vi "Teleop.vi"(10 "Match Info":T1={"Autonomous Elapsed Seconds"=0.0, "TeleOp Elapsed Seconds"=0.0, "Disabled Elapsed Seconds"=0.0, "Visited Autonomous"=FALSE, "Visited TeleOp"=FALSE, "Visited Disabled"=FALSE, "Autonomous Settings"={"Autonomous Style"=enum."Independent", "VI Refnum"=refnum}}, 11 "Call Context":T2) -> ()   [LabVIEW 2015]
doc: "This VI is called for each TeleOp packet received from the DS where the robot is not disabled. It is often used to read from the joysticks and update I/O or to update setpoints for timed control loops. It should complete and return within 20 milliseconds or it may miss DS packets."
uses:
  <vilib>/Rock Robotics/WPI/DriverStation/WPI_DriverStationDerivedRobotMode.ctl
  <vilib>/Rock Robotics/WPI/DriverStation/WPI_DriverStationMatch Info.ctl
  <vilib>/Rock Robotics/WPI/Solenoid/WPI_SolenoidValue.ctl
  <vilib>/Rock Robotics/WPI/Utilities/WPI_GetSetVariantRefNum.vi
  <vilib>/Rock Robotics/Network Tables/NT Write Boolean Array.vi
  <vilib>/Rock Robotics/Network Tables/NT Write Numeric Array.vi
  <vilib>/Rock Robotics/Network Tables/NT Read Boolean.vi
  <vilib>/Rock Robotics/Network Tables/NT Read Number.vi
  <vilib>/Rock Robotics/WPI/Solenoid/WPI_SolenoidSetEnum.vi
  <vilib>/Rock Robotics/Network Tables/NT Write Number.vi
panel:
  out "Compressor Running":bool
  out "Enabled":bool
  out "Sample Slider 0":dbl(slide) scale=0.0..5.0
  out "Sample Boolean 1":bool
  out "Sample Boolean 0":bool
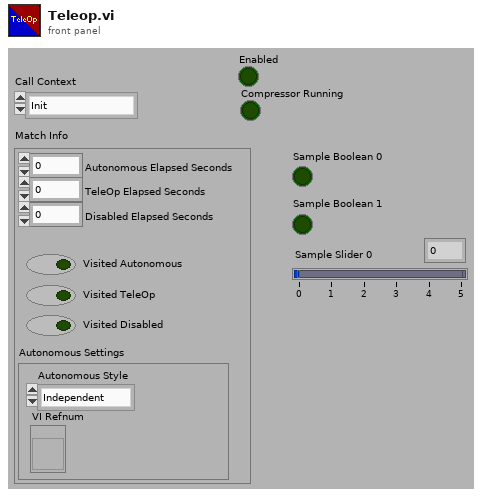
[diagram p1: front panel]
types:
  T1 = typedef "WPI_DriverStationMatch Info.ctl" = cluster{"Autonomous Elapsed Seconds":dbl, "TeleOp Elapsed Seconds":dbl, "Disabled Elapsed Seconds":dbl, "Visited Autonomous":bool, "Visited TeleOp":bool, "Visited Disabled":bool, "Autonomous Settings":cluster{"Autonomous Style":enum16{"Iterative", "Independent"}, "VI Refnum":refnum<vi>}}
  T2 = typedef "WPI_DriverStationDerivedRobotMode.ctl" = enum16{"Init", "Execute", "Stop"}
  T3 = typedef "WPI_CompressorDevRef.ctl" = cluster{"DevStatus":errorcluster, "Pneumatics Control Module":u8}
  T4 = typedef "WPI_RobotDriveDevRef.ctl" = cluster{"DevStatus":errorcluster, "Motors[]":T5[], "Square Inputs":bool, "Max Output":dbl}
  T5 = typedef "WPI_MotorControlDeviceRef.ctl" = cluster{"DeviceStatus":errorcluster, "Type":T6, "PWM":cluster{"PWM Channel":T7, "DeadBand":T8}, "CAN":cluster{"Device Number":u8, "Control Mode":T9, "Semaphore":T10, "Max Vout":dbl, "TalonSRX Control Mode":T11}, "Invert":bool}
  T6 = typedef "WPI_MotorControlType.ctl" = enum16{"PWM", "CAN", "CANTalonSRX"}
  T7 = typedef "FPGA_DIOPWMChannel.ctl" = enum8{"PWM 0", "PWM 1", "PWM 2", "PWM 3", "PWM 4", "PWM 5", "PWM 6", "PWM 7", "PWM 8", "PWM 9", "PWM MXP 0", "PWM MXP 1", "PWM MXP 2", "PWM MXP 3", "PWM MXP 4", "PWM MXP 5", "PWM MXP 6", "PWM MXP 7", "PWM MXP 8", "PWM MXP 9", "Invalid"}
  T8 = typedef "WPI_PWMDeadband.ctl" = cluster{"Name":string, "maxPositivePwm":i32, "minPositivePwm":i32, "centerPwm":i32, "maxNegativePwm":i32, "minNegativePwm":i32, "angularRange":u16}
  T9 = typedef "WPI_CANJaguar_ControlMode.ctl" = enum8{"Percent VBus", "Current", "Speed", "Position", "Voltage"}
  T10 = typedef "Semaphore RefNum" = refnum<k1>
  T11 = typedef "WPI_CANTalonSRX_APIControlMode.ctl" = enum8{"Percent VBus", "Speed", "Position", "Slave", "Unchanged / Invalid", "Voltage Compensation", "Current", "Motion Profile"}
  T12 = typedef "WPI_JoystickDevRef.ctl" = cluster{"Device":T13}
  T13 = typedef "WPI_JoystickDeviceEnum.ctl" = enum16{"USB 0", "USB 1", "USB 2", "USB 3", "USB 4", "USB 5"}
  T14 = typedef "WPI_SolenoidValue.ctl" = enum16{"Off", "On", "Forward", "Reverse"}
  T15 = typedef "WPI_SolenoidDevRef.ctl" = cluster{"DevStatus":errorcluster, "Pneumatics Control Module":u8, "Forward Solenoid Channel":T16, "Reverse Solenoid Channel":T16}
  T16 = typedef "WPI_SolenoidChannel.ctl" = enum8{"Solenoid 0", "Solenoid 1", "Solenoid 2", "Solenoid 3", "Solenoid 4", "Solenoid 5", "Solenoid 6", "Solenoid 7", "Invalid"}
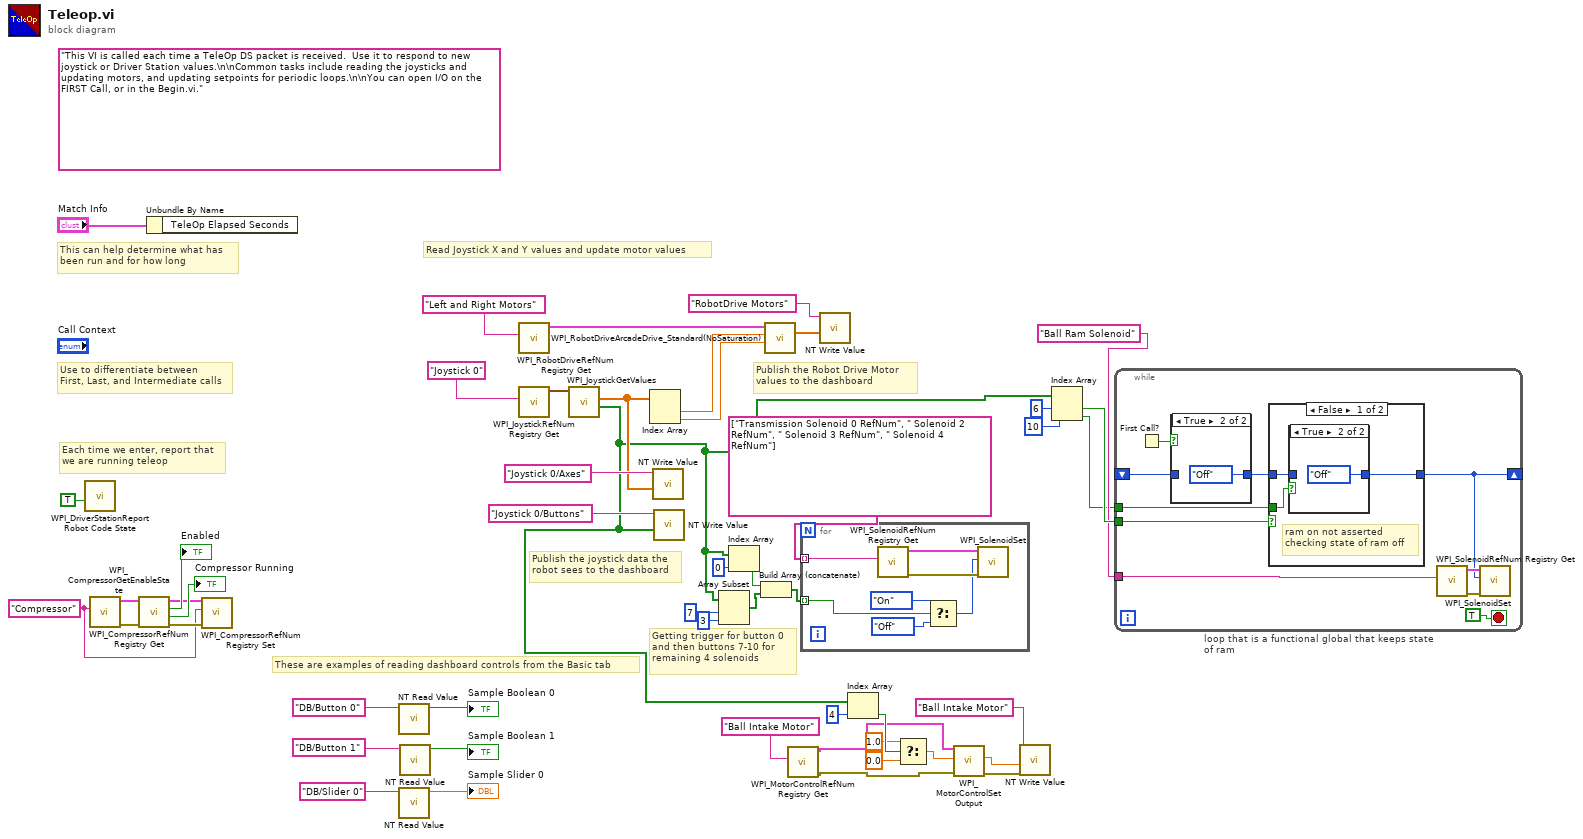
[diagram p0: block diagram]
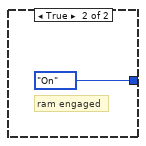
[diagram p4: hidden frame]
diagram:
  w25 = "Compressor" ("refnum name")
  (unwired) "This VI is called each time a TeleOp DS packet is received.  Use it to respond to new joystick or Driver Station values.\n\nCommon tasks include reading the joysticks and updating motors, and updating setpoints for periodic loops.\n\nYou can open I/O on the FIRST Call, or in the Begin.vi."
  # "Getting trigger for button 0\nand then buttons 7-10 for\nremaining 4 solenoids"
  # "These are examples of reading dashboard controls from the Basic tab"
  # "Publish the Robot Drive Motor\nvalues to the dashboard"
  # "Publish the joystick data the\nrobot sees to the dashboard"
  # "Each time we enter, report that\nwe are running teleop"
  # "Use to differentiate between\nFirst, Last, and Intermediate calls"
  # "This can help determine what has\nbeen run and for how long"
  # "Read Joystick X and Y values and update motor values"
  n1 = call <vilib>:"WPI_DriverStationReport Robot Code State.vi"("TeleOp"=TRUE ("Autonomous")) -> ()  [unwired: 10 in, 1 out]
  n2 = call <vilib>:"WPI_CompressorRefNum Registry Get.vi"("refnum name"=w25) -> ("error out"=w31:errorcluster, "CompressorDevRef"=w30:T3)  [unwired: 9 in]
  n3 = call <vilib>:"WPI_CompressorGetEnableState.vi"("error in (no error)"=w31, "CompressorDevRef"=w30) -> ("error out"=w26:errorcluster, "Compressor Running"=→"Compressor Running":bool, "Enabled"=→"Enabled":bool, "CompressorDevRef"=w27:T3)  [unwired: 6 in]
  n4 = Unbundle By Name("Match Info") -> ()  [unwired: 1 out]
  n5 = call <vilib>:"WPI_CompressorRefNum Registry Set.vi"("error in (no error)"=w26, "refnum name"=w25, "CompressorDevRef"=w27) -> ()  [unwired: 7 in, 2 out]
  n6 = call-poly <vilib>:"NT Read Value.vi"("Name"="DB/Button 0" ("refnum name")) -> ("Boolean"=→"Sample Boolean 0":bool)  [unwired: 9 in, 1 out]
  n7 = call-poly <vilib>:"NT Read Value.vi"("Name"="DB/Slider 0" ("refnum name")) -> ("Numeric"=→"Sample Slider 0":dbl)  [unwired: 9 in, 1 out]
  n8 = call-poly <vilib>:"NT Read Value.vi"("Name"="DB/Button 1" ("refnum name")) -> ("Boolean"=→"Sample Boolean 1":bool)  [unwired: 9 in, 1 out]
  n9 = call <vilib>:"WPI_RobotDriveRefNum Registry Get.vi"("refnum name"="Left and Right Motors") -> ("RobotDriveDevRef"=w48:T4)  [unwired: 1 in, 9 out]
  n10 = call <vilib>:"WPI_JoystickRefNum Registry Get.vi"("refnum name"="Joystick 0") -> ("JoystickDevRef"=w45:T12)  [unwired: 1 in, 9 out]
  n11 = call <vilib>:"WPI_JoystickGetValues.vi"("JoystickDevRef"=w45) -> ("Buttons"=w4:bool[], "Axes"=w40:dbl[])  [unwired: 6 in, 3 out]
  n12 = Index Array(array=w40) -> (element #1=w47:dbl, element #2=w43:dbl)  [unwired: 2 in]
  n13 = call-poly <vilib>:"NT Write Value.vi"("Numeric Array"=w40, "Name"="Joystick 0/Axes") -> ()  [unwired: 9 in, 1 out]
  n14 = call-poly <vilib>:"NT Write Value.vi"("Boolean Array"=w4, "Name"="Joystick 0/Buttons") -> ()  [unwired: 9 in, 1 out]
  n15 = Array Subset(array=w4, index=7, length=3) -> (w19:bool[])
  n16 = Index Array(array=w4, index=0) -> (element=w20:bool)
  n17 = Build Array (concatenate)(w20, w19) -> (w18:bool[])
  n18 = call <vilib>:"WPI_RobotDriveArcadeDrive_Standard(NoSaturation).vi"("Y axis value"=w43, "X axis value"=w47, "RobotDriveDevRef"=w48) -> ("Motor Values"=w33:dbl[])  [unwired: 1 in, 7 out]
  n19 = call <vilib>:"WPI_MotorControlRefNum Registry Get.vi"("refnum name"="Ball Intake Motor") -> ("error out"=w9:errorcluster, "MotorControlDevRef"=w8:T5)  [unwired: 9 in]
  n20 = for {
    tunnel: w18 -> [w51] mode=indexing
    tunnel: string[] ["Transmission Solenoid 0 RefNum", " Solenoid 2 RefNum", " Solenoid 3 RefNum", " Solenoid 4 RefNum"] -> [w52] mode=indexing
    n21 = call <vilib>:"WPI_SolenoidRefNum Registry Get.vi"("refnum name"=w52) -> ("error out"=w57:errorcluster, "SolenoidDevRef"=w56:T15)  [unwired: 9 in]
    n22 = Select(t=WPI_SolenoidValue."On" ("Value"), s=w51, f=WPI_SolenoidValue."Off" ("Value")) -> (s? t:f=w53:T14)
    n23 = call-poly <vilib>:"WPI_SolenoidSet.vi"("error in (no error)"=w57, "Value"=w53, "SolenoidDevRef"=w56) -> ()  [unwired: 7 in, 2 out]
  }
  n24 = call-poly <vilib>:"NT Write Value.vi"("Numeric Array"=w33, "Name"="RobotDrive Motors") -> ()  [unwired: 9 in, 1 out]
  n25 = Index Array(array=w4, index=4) -> (element=w16:bool)
  n26 = Select(t=1.0, s=w16, f=0.0) -> (s? t:f=w15:dbl)
  n27 = call <vilib>:"WPI_MotorControlSetOutput.vi"("error in (no error)"=w9, "Output"=w15, "MotorControlDevRef"=w8) -> ("error out"=w12:errorcluster, "Motor Output"=w10:dbl)  [unwired: 6 in, 1 out]
  n28 = call-poly <vilib>:"NT Write Value.vi"("error in"=w12, "Numeric"=w10, "Name"="Ball Intake Motor") -> ()  [unwired: 8 in, 1 out]
  n29 = Index Array(array=w4, index #1=6 ("index"), index #2=10 ("index")) -> (element #1=w5:bool, element #2=w1:bool)
  n30 = while "loop that is a functional global that keeps state of ram" {
    shift-right: [w63] -> _
    shift-left: _ -> [w59]
    tunnel: w5 -> [w64]
    tunnel: w1 -> [w62]
    tunnel: "Ball Ram Solenoid" ("refnum name") -> [w61]
    stop <- TRUE stop-if-true
    n31 = First Call?() -> (First Call?: T/F=w60:bool)
    n32 = case shown="True" w60 {
      tunnel: w59 -> [w68 _]
      tunnel: [w68 WPI_SolenoidValue."Off" ("Value")] -> w58
      frame False {
      }
      frame True {
      }
    }
    n33 = case shown="False" w64 {
      tunnel: [w71 WPI_SolenoidValue."On" ("Value")] -> w63
      tunnel: w58 -> [w70 _]
      tunnel: w62 -> [w72 _]
      frame False {
        # "ram on not asserted\nchecking state of ram off"
        n34 = case shown="True" w72 {
          tunnel: [w73 WPI_SolenoidValue."Off" ("Value")] -> w71
          tunnel: w70 -> [w73 _]
          frame False {
          }
          frame True {
          }
        }
      }
      frame True {
        # "ram engaged"
      }
    }
    n35 = call <vilib>:"WPI_SolenoidRefNum Registry Get.vi"("refnum name"=w61) -> ("error out"=w67:errorcluster, "SolenoidDevRef"=w66:T15)  [unwired: 9 in]
    n36 = call-poly <vilib>:"WPI_SolenoidSet.vi"("error in (no error)"=w67, "Value"=w63, "SolenoidDevRef"=w66) -> ()  [unwired: 7 in, 2 out]
  }
